vi "sc5511a_set_synth_mode.vi"(0 "deviceHandle":u32 format="%.0x", 1 "Harmonic Spur Suppression":u8(ring) items=["Enabled", "Disable"], 2 "loop gain":u8(ring) items=["Normal", "Low"], 3 "lock mode":u8(ring) items=["Harmonic Loop", "Fractional Loop"], 5 "error in":errorcluster) -> (14 "deviceHandle":u32 format="%.0x", 19 "error out":errorcluster)   [LabVIEW 2010]
uses:
  sc5511a.dll
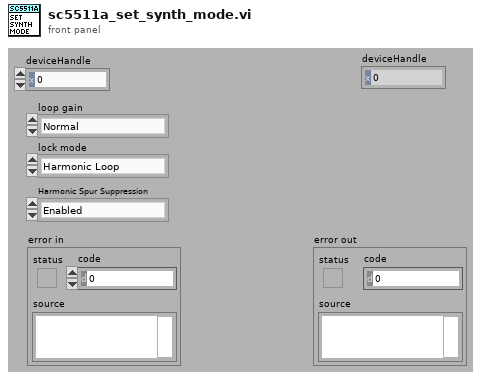
[diagram p1: front panel]
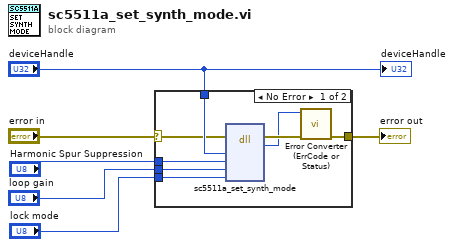
[diagram p0: block diagram]
diagram:
  n1 = case shown="No Error" "error in" {
    selector: "error in" -> [w9 w15]
    tunnel: [w14 w15] -> w6
    tunnel: "deviceHandle" -> [w11 _]
    tunnel: "lock mode" -> [w10 _]
    tunnel: "loop gain" -> [w8 _]
    tunnel: "Harmonic Spur Suppression" -> [w7 _]
    frame No Error {
      n2 = dll-call lib="sc5511a.dll" fn="sc5511a_set_synth_mode"(error in=w9, "deviceHandle"=w11, "disable_spur_suppression"=w7, "loop_gain"=w8, "lock_mode"=w10) -> (error out=w13:errorcluster, "return type"=w12:i32)  [unwired: 6 in, 1 out]
      n3 = call "Error Converter (ErrCode or Status).vi"("error in (no error)"=w13, "error code"=w12) -> ("error out"=w14:errorcluster)  [unwired: 9 in]
    }
    frame Error {
    }
  }
  "error out" <- w6
  "deviceHandle" <- "deviceHandle"
